vi "Encoders Remove Outliers.vi"(0 "array":T1(array[cluster])) -> (1 "Mean Distance":dbl, 2 "Mean Rate":dbl)   [LabVIEW 2014]
uses:
  <vilib>/gmath/NI_Gmath.lvlib
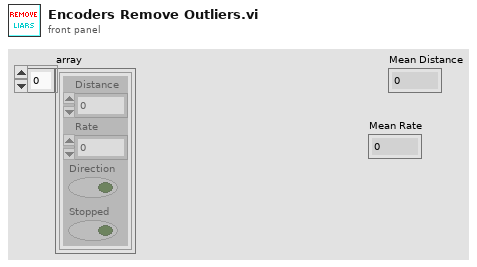
[diagram p1: front panel]
types:
  T1 = cluster{"Distance":dbl, "Rate":dbl, "Direction":bool, "Stopped":bool}[]
  T2 = enum16{"arithmetic", "geometric", "harmonic", "trimmed", "median"}
  T3 = cluster{"Distance":dbl, "Rate":dbl, "Direction":bool, "Stopped":bool}
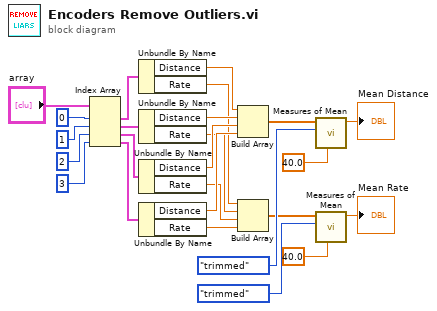
[diagram p0: block diagram]
diagram:
  n1 = Index Array(array="array", index #1=0 ("index"), index #2=1 ("index"), index #3=2 ("index"), index #4=3 ("index")) -> (element #1=w17:T3, element #2=w16:T3, element #3=w15:T3, element #4=w14:T3)
  n2 = Unbundle By Name(w17) -> ("Distance"=w10:dbl, "Rate"=w5:dbl)
  n3 = Unbundle By Name(w16) -> ("Distance"=w9:dbl, "Rate"=w4:dbl)
  n4 = Unbundle By Name(w15) -> ("Distance"=w8:dbl, "Rate"=w3:dbl)
  n5 = Unbundle By Name(w14) -> ("Distance"=w7:dbl, "Rate"=w2:dbl)
  n6 = Build Array(w10, w9, w8, w7) -> (w6:dbl[])
  n7 = Build Array(w5, w4, w3, w2) -> (w1:dbl[])
  n8 = call <vilib>:"Measures of Mean.vi"("percent (trim)"=40.0, "type"=T2."trimmed", "x array"=w6) -> ("mean value"=→"Mean Distance":dbl)  [unwired: 7 in, 1 out]
  n9 = call <vilib>:"Measures of Mean.vi"("percent (trim)"=40.0, "type"=T2."trimmed", "x array"=w1) -> ("mean value"=→"Mean Rate":dbl)  [unwired: 7 in, 1 out]
